vi "test3-RegisterUnregister_Queue.vi"(8 "error in (no error)":errorcluster, 11 "TestCase in":refnum<class "testcase-CSMGlobalLog.lvclass">) -> (0 "error out":errorcluster, 3 "TestCase out":refnum<class "testcase-CSMGlobalLog.lvclass">)   [LabVIEW 2017, in "testcase-CSMGlobalLog.lvclass"]
uses:
  testcase-CSMGlobalLog.lvclass
  testcase-CSMGlobalLog.lvclass/testcase-CSMGlobalLog.ctl
  e676bdd4-339a-4016-80a7-73cacdf207a1.vi
  663c4efc-b474-423a-ba8f-9e42956192f1.vi
  <vilib>/addons/_JKI Toolkits/VI Tester/TestCase.llb/TestCase.lvclass
  src/user.lib/_NEVSTOP/Communicable State Machine(CSM)/Utility/Periodic String Filter Setting.ctl
  src/user.lib/_NEVSTOP/Communicable State Machine(CSM)/Communicable State Machine.lvlib
  C:/Program Files (x86)/National Instruments/LabVIEW 2017/vi.lib/addons/_JKI Toolkits/VI Tester/TestCase.llb/TestCase.lvclass
panel:
  out "String cache total":string
  out "LoopCount":i32
  out "String Cache Each Loop":string
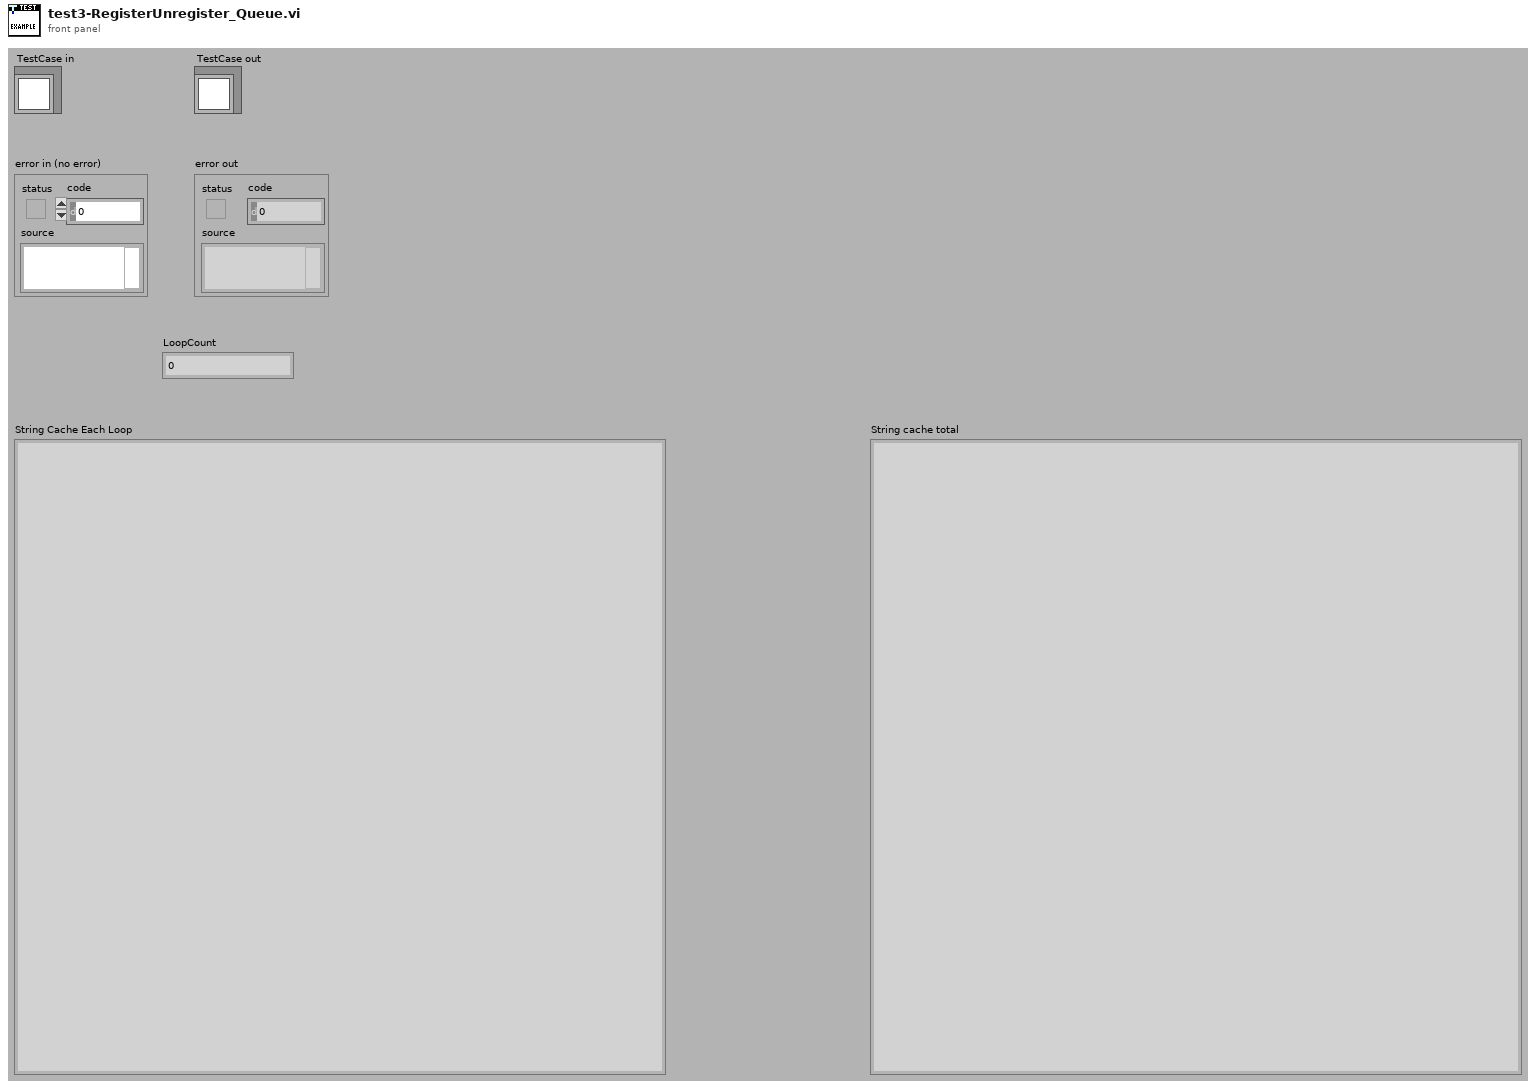
[diagram p1: front panel]
types:
  T1 = typedef "Communicable State Machine.lvlib/Periodic String Filter Setting.ctl" = cluster{"threashold(#/s)":dbl, "Check Peroid(s)":dbl}
  T2 = typedef "Communicable State Machine.lvlib/_CSM_GlobalLog_MSG.ctl" = cluster{"Name (\"\" to Use UUID)":string, "Current State":string, "Arguments":string, "Source Message":T3, "Source Module":string, "Complete(T)/Start(F)":bool, "LogType":T4, "Time Stamp":timestamp}
  T3 = typedef "Communicable State Machine.lvlib/_CSM_Response Source Message.ctl" = cluster{"‘State":string, "’Arguments":string, "’Error":errorcluster}
  T4 = typedef "Communicable State Machine.lvlib/_CSM_GlobalLog_MSG_TYPE.ctl" = enum16{"User Log", "State Change", "Status", "Interrupt", "Register", "Unregister", "Error Log", "Module Created", "Module Destroyed", "Async Message", "No-Rep Async Message", "Sync Message"}
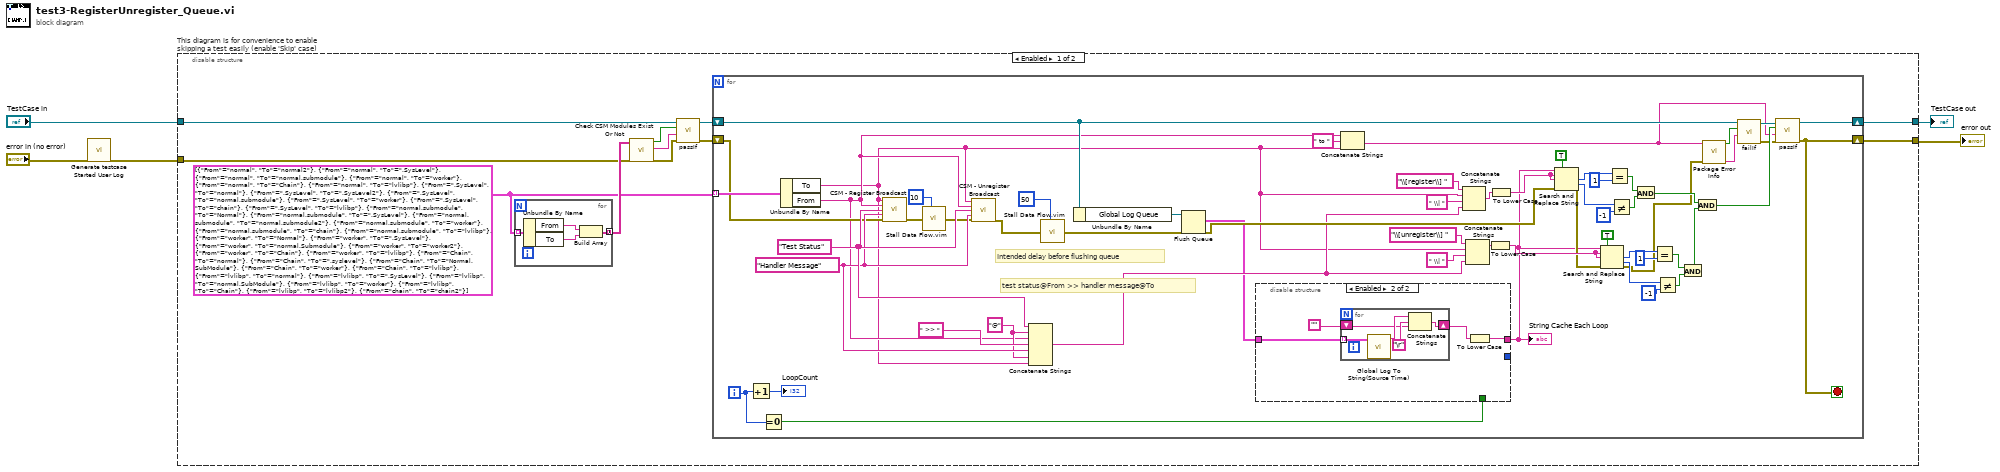
[diagram p0: block diagram]
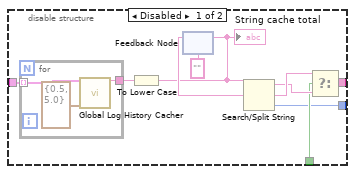
[diagram p2: hidden frame]
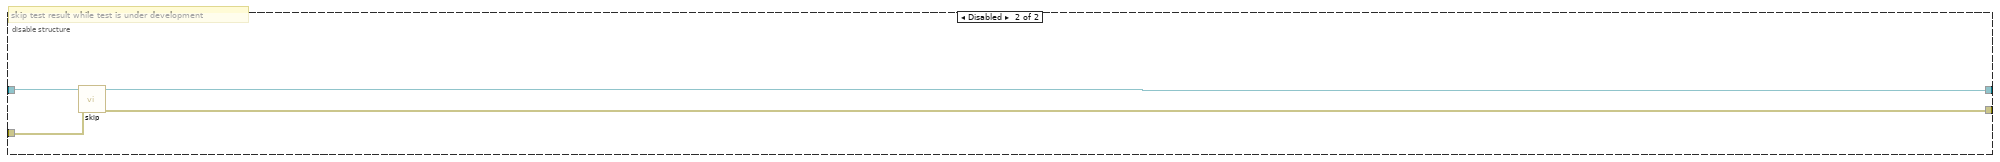
[diagram p3: hidden frame]
diagram:
  n1 = call "Generate testcase Started User Log.vi"("Error In"="error in (no error)") -> ("error out"=w1:errorcluster)  [unwired: 10 in]
  n2 = disable-structure "This diagram is for convenience to enable skipping a test easily (enable 'Skip' case)" shown="Enabled" {
    disable-tunnel: "TestCase in" -> [w9 w104]
    disable-tunnel: [w15 w102] -> w2
    disable-tunnel: [w16 w103] -> w4
    disable-tunnel: w1 -> [w6 w101]
    frame Enabled {
      w10 = cluster{"From":string, "To":string}[] [{"From"="normal", "To"="normal2"}, {"From"="normal", "To"=".SysLevel"}, {"From"="normal", "To"="normal.submodule"}, {"From"="normal", "To"="worker"}, {"From"="normal", "To"="Chain"}, {"From"="normal", "To"="lvlibp"}, {"From"=".SysLevel", "To"="normal"}, {"From"=".SysLevel", "To"=".SysLevel2"}, {"From"=".SysLevel", "To"="normal.submodule"}, {"From"=".SysLevel", "To"="worker"}, {"From"=".SysLevel", "To"="chain"}, {"From"=".SysLevel", "To"="lvlibp"}, {"From"="normal.submodule", "To"="Normal"}, {"From"="normal.submodule", "To"=".SysLevel"}, {"From"="normal.submodule", "To"="normal.submodule2"}, {"From"="normal.submodule", "To"="worker"}, {"From"="normal.submodule", "To"="chain"}, {"From"="normal.submodule", "To"="lvlibp"}, {"From"="worker", "To"="Normal"}, {"From"="worker", "To"=".SysLevel"}, {"From"="worker", "To"="normal.Submodule"}, {"From"="worker", "To"="worker2"}, {"From"="worker", "To"="Chain"}, {"From"="worker", "To"="lvlibp"}, {"From"="Chain", "To"="normal"}, {"From"="Chain", "To"=".syslevel"}, {"From"="Chain", "To"="Normal.SubModule"}, {"From"="Chain", "To"="worker"}, {"From"="Chain", "To"="lvlibp"}, {"From"="lvlibp", "To"="normal"}, {"From"="lvlibp", "To"=".SysLevel"}, {"From"="lvlibp", "To"="normal.SubModule"}, {"From"="lvlibp", "To"="worker"}, {"From"="lvlibp", "To"="Chain"}, {"From"="lvlibp", "To"="lvlibp2"}, {"From"="chain", "To"="chain2"}]
      n3 = for {
        tunnel: w10 -> [w20] mode=indexing
        tunnel: [w17] -> w13 mode=concatenating
        n4 = Unbundle By Name(w20) -> ("From"=w19:string, "To"=w18:string)
        n5 = Build Array(w19, w18) -> (w17:string[])
      }
      n6 = call "Check CSM Modules Exist Or Not.vi"("error in"=w6, "CSM names in"=w13) -> ("error out"=w11:errorcluster, "Debug string"=w12:string, "All Modules Exist?"=w14:bool)  [unwired: 7 in]
      n7 = call-dynamic "passIf.vi"("error in (no error)"=w11, "message (\"\")"=w12, "pass"=w14, "TestCase in"=w9) -> ("error out"=w7:errorcluster, "TestCase out"=w8:refnum<class "testcase-CSMGlobalLog.lvclass">)  [unwired: 6 in]
      n8 = for {
        tunnel: w10 -> [w49] mode=indexing
        shift-right: [w42] -> w16
        shift-left: w7 -> [w34]
        shift-right: [w78] -> w15
        shift-left: w8 -> [w31]
        i -> [w37]
        stop <- w42 stop-if-true
        w45 = "@" ("Trigger")
        w46 = "Handler Message" ("API (If \"\", Same as Trigger)")
        w47 = "Test Status" ("Trigger")
        # "Intended delay before flushing queue"
        # "test status@From >> handler message@To"
        n9 = Increment(x=w37) -> (x+1=→"LoopCount":i32)
        n10 = Equal To 0?(x=w37) -> (x = 0?=w36:bool)
        n11 = Unbundle By Name(w49) -> ("To"=w26:string, "From"=w27:string)
        n12 = call "CSM - Register Broadcast.vi"("CSM Name(Empty for Broadcast Event)"=w26, "Source CSM Name (* as Default)"=w27, "Trigger"=w47, "API (If \"\", Same as Trigger)"=w46, "Error In"=w34) -> ("error out"=w23:errorcluster)  [unwired: 9 in, 1 out]
        n13 = call "Stall Data Flow.vim"("value in"=w23, "milliseconds to wait"=u32 10) -> ("value out"=w22:errorcluster)  [unwired: 1 out]
        n14 = call "CSM - Unregister Broadcast.vi"("CSM Name(Empty for Broadcast Event)"=w26, "Source CSM Name (* as Default)"=w27, "Trigger"=w47, "API (\"*\" as Default)"=w46, "Error In"=w22) -> ("error out"=w41:errorcluster)  [unwired: 9 in, 1 out]
        n15 = Concatenate Strings(w47, w45, w27, " >> " ("string"), w46, w45, w26) -> (w44:string)
        n16 = call "Stall Data Flow.vim"("value in"=w41, "milliseconds to wait"=u32 50) -> ("value out"=w40:errorcluster)  [unwired: 1 out]
        n17 = Unbundle By Name(w31) -> ("Global Log Queue"=w77:refnum<queue>)
        n18 = Flush Queue(queue=w77, error in (no error)=w40) -> (remaining elements=w35:T2[], error out=w55:errorcluster)  [unwired: 1 out]
        n19 = disable-structure shown="Enabled" {
          disable-tunnel: [w82 w92] -> w38
          disable-tunnel: w36 -> [w81 _]
          disable-tunnel: [w80 _] -> _
          disable-tunnel: w35 -> [w79 w94]
          frame Disabled {
            n20 = for {
              tunnel: w79 -> [w91] mode=indexing
              tunnel: [w90] -> w88
              n21 = call "Global Log History Cacher.vi"("Global Log Data"=w91, "Settings"=T1 {"threashold(#/s)"=0.5, "Check Peroid(s)"=5.0}) -> ("String Cache"=w90:string)  [unwired: 13 in]
            }
            n22 = To Lower Case(string=w88) -> (all lower case string=w83:string)
            "String cache total" <- w83
            n23 = feedback #1("") -> (w87:string)
            n24 = feedback-in #1(w83) -> ()
            n25 = Search/Split String(string=w83, search string/char (-)=w87) -> (substring before match=w84:string, match + rest of string=w85:string, offset of match=w80:i32)  [unwired: 1 in]
            n26 = Select(t=w85, s=w81, f=w84) -> (s? t:f=w82:string)
          }
          frame Enabled {
            n27 = for {
              tunnel: w94 -> [w100] mode=indexing
              shift-right: [w96] -> w93
              shift-left: "" -> [w97]
              n28 = call "Global Log To String(Source Time).vi"("Log"=w100) -> ("Log String"=w99:string)  [unwired: 9 in]
              n29 = Concatenate Strings(w99, "\r", w97) -> (w96:string)
            }
            n30 = To Lower Case(string=w93) -> (all lower case string=w92:string)
          }
        }
        "String Cache Each Loop" <- w38
        n31 = Concatenate Strings(w27, " to " ("string"), w26) -> (w24:string)
        n32 = Concatenate Strings("\\[register\\] " ("regular expression"), w26, " \\| " ("string"), w44) -> (w72:string)
        n33 = Concatenate Strings("\\[unregister\\] " ("regular expression"), w26, " \\| " ("string"), w44) -> (w74:string)
        n34 = To Lower Case(string=w74) -> (all lower case string=w58:string)
        n35 = To Lower Case(string=w72) -> (all lower case string=w70:string)
        n36 = Search and Replace String(replace all?=TRUE ("replace all? (F)"), input string=w38, search string=w70, replace string=w70, error in=w55) -> (number of replacements=w69:i32, offset past replacement=w68:i32, error out=w57:errorcluster)  [unwired: 3 in, 1 out]
        n37 = Search and Replace String(replace all?=TRUE ("replace all? (F)"), input string=w38, search string=w58, replace string=w58, error in=w57) -> (number of replacements=w60:i32, offset past replacement=w61:i32, error out=w28:errorcluster)  [unwired: 3 in, 1 out]
        n38 = Equal?(x=w69, y=1) -> (x = y?=w66:bool)
        n39 = Not Equal?(x=w68, y=-1) -> (x != y?=w65:bool)
        n40 = And(x=w66, y=w65) -> (x .and. y?=w50:bool)
        n41 = Equal?(x=w60, y=1) -> (x = y?=w63:bool)
        n42 = Not Equal?(x=w61, y=-1) -> (x != y?=w64:bool)
        n43 = And(x=w63, y=w64) -> (x .and. y?=w56:bool)
        n44 = And(x=w50, y=w56) -> (x .and. y?=w43:bool)
        n45 = call "Package Error Info.vi"("error in"=w28, "String in"=w24) -> ("packed error info out"=w32:string, "error status"=w33:bool)  [unwired: 8 in]
        n46 = call-dynamic "failIf.vi"("message (\"\")"=w32, "fail"=w33, "TestCase in"=w31) -> ("error out"=w29:errorcluster, "TestCase out"=w30:refnum<class "testcase-CSMGlobalLog.lvclass">)  [unwired: 7 in]
        n47 = call-dynamic "passIf.vi"("error in (no error)"=w29, "message (\"\")"=w24, "pass"=w43, "TestCase in"=w30) -> ("error out"=w42:errorcluster, "TestCase out"=w78:refnum<class "testcase-CSMGlobalLog.lvclass">)  [unwired: 6 in]
      }
    }
    frame Disabled {
      # "skip test result while test is under development"
      n48 = call <vilib>:"skip.vi"("error in (no error)"=w101, "TestCase in"=w104) -> ("error out"=w103:errorcluster, "TestCase out"=w102:refnum<class "testcase-CSMGlobalLog.lvclass">)  [unwired: 8 in]
    }
  }
  "error out" <- w4
  "TestCase out" <- w2
